vi "HMI Connect Streams.vi"(11 "Target Address":string="172.22.11.2") -> (0 "error out":errorcluster, 2 "reader endpoint":refnum<k21>, 3 "writer endpoint":refnum<k21>)   [LabVIEW 2021]
uses:
  GV/HMI GV.vi
panel:
  in  "timeout in ms (-1)":i32=500
  in  "error in":errorcluster
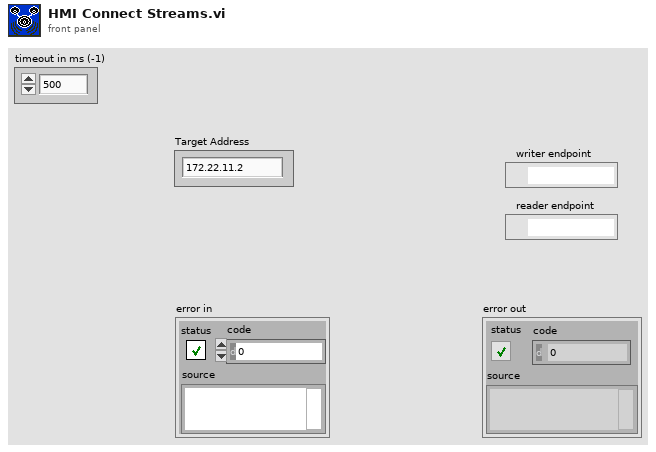
[diagram p1: front panel]
types:
  T1 = cluster{"Message":string, "Message Data":variant}
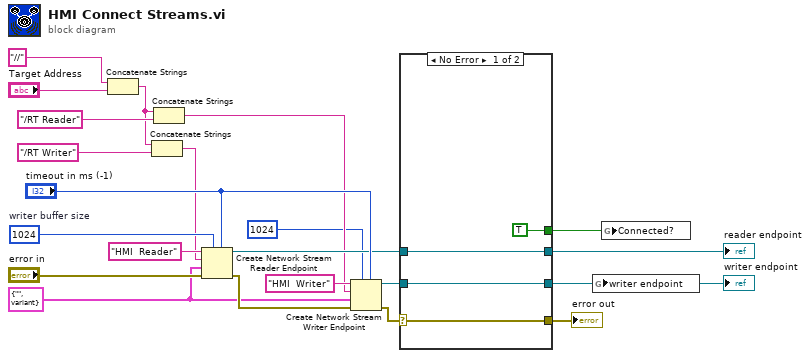
[diagram p0: block diagram]
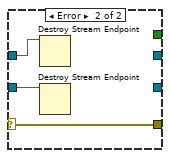
[diagram p2: hidden frame]
diagram:
  w19 = 1024  # writer buffer size
  w3 = T1 {"Message"="", "Message Data"=variant} ("Message Cluster")
  n1 = Concatenate Strings("//" ("writer url"), "Target Address") -> (w12:string)
  n2 = Concatenate Strings(w12, "/RT Writer" ("writer url")) -> (w6:string)
  n3 = Concatenate Strings(w12, "/RT Reader" ("writer url")) -> (w5:string)
  n4 = Create Network Stream Reader Endpoint(5:"timeout in ms (-1)", 7:w19, 8:"error in", 9:w3, 10:w6, 11:"HMI  Reader" ("writer name")) -> (0:w8:errorcluster, 3:w16:refnum<k21>)  [unwired: 1 in]
  n5 = Create Network Stream Writer Endpoint(5:"timeout in ms (-1)", 7:1024 ("writer buffer size"), 8:w8, 9:w3, 10:w5, 11:"HMI  Writer" ("reader name")) -> (0:w18:errorcluster, 3:w15:refnum<k21>)  [unwired: 1 in]
  n6 = case shown="No Error" w18 {
    selector: w18 -> [w26 w27]
    tunnel: [w26 w27] -> w17
    tunnel: w16 -> [w25 w29]
    tunnel: [w25 _] -> w9
    tunnel: w15 -> [w24 w28]
    tunnel: [w24 _] -> w2
    tunnel: [TRUE _] -> w1
    frame No Error {
    }
    frame Error {
      n7 = Destroy Stream Endpoint(11:w29) -> ()  [unwired: 1 in, 1 out]
      n8 = Destroy Stream Endpoint(11:w28) -> ()  [unwired: 1 in, 1 out]
    }
  }
  "error out" <- w17
  "reader endpoint" <- w9
  "writer endpoint" <- w2
  n9 = global write "HMI GV.vi" "writer endpoint"(w2) -> ()
  n10 = global write "HMI GV.vi" "Connected?"(w1) -> ()
